vi "ReadSimbolValue.vi"(8 "error in (no error)":errorcluster, 10 "name":string, 11 "TCatAdsNet in":refnum<class "AdsNET.lvclass">) -> (0 "error out":errorcluster, 1 "Datatype":i32, 2 "Value":string, 3 "TCatAdsNet out":refnum<class "AdsNET.lvclass">, 4 "Elapsed Time (ms)":u32)   [LabVIEW 2016, in "TCatAdsNet.lvlib" / "AdsNET.lvclass"]
uses:
  AdsNET.lvclass
  AdsNET.lvclass/AdsNET.ctl
  C:/Users/Maurizio/Projects/twincat-lv-ads-library/TCatAdsNet Library/TwinCAT.Ads.dll
  TwinCAT.Ads.dll
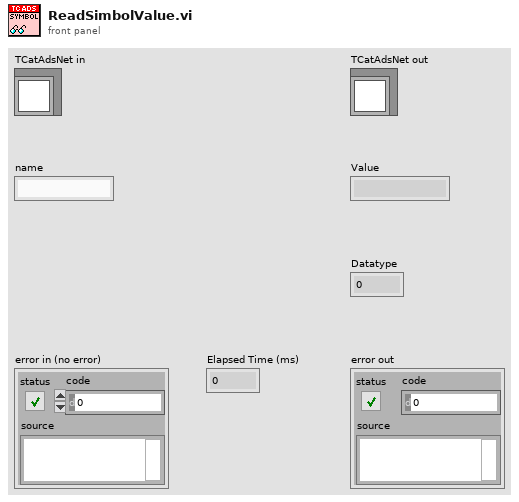
[diagram p1: front panel]
types:
  T1 = cluster{"Name":string, "IndexGroup":i64, "IndexOffset":i64, "Size":i32, "Type":string, "Datatype":i32, "Comment":string}
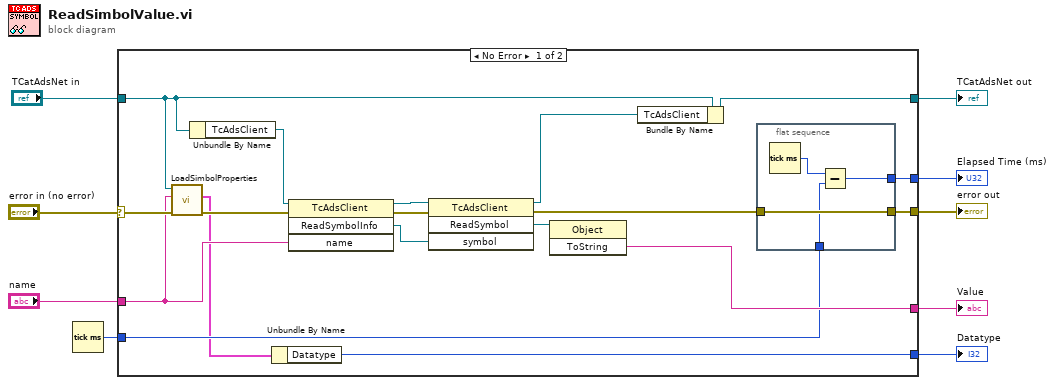
[diagram p0: block diagram]
diagram:
  n1 = Tick Count (ms)() -> (millisecond timer value=w3:u32)
  n2 = case shown="No Error" "error in (no error)" {
    selector: "error in (no error)" -> [w15 w32]
    tunnel: [w18 w32] -> w9
    tunnel: "TCatAdsNet in" -> [w12 w33]
    tunnel: "name" -> [w13 _]
    tunnel: [w22 _] -> w6
    tunnel: [w21 w33] -> w5
    tunnel: w3 -> [w17 _]
    tunnel: [w16 _] -> w2
    tunnel: [w10 _] -> w1
    frame No Error {
      n3 = call "LoadSimbolProperties.vi"("error in (no error)"=w15, "name"=w13, "TCatAdsNet in"=w12) -> ("error out"=w14:errorcluster, "SymbolProperties"=w11:T1)  [unwired: 5 in, 2 out]
      n4 = Unbundle By Name(w12) -> ("TcAdsClient"=w23:refnum<k24>)
      n5 = Unbundle By Name(w11) -> ("Datatype"=w10:i32)
      n6 = invoke class="TcAdsClient" method="ReadSymbolInfo"(reference=w23, error in=w14, "name"=w13) -> (reference out=w26:refnum<k24>, error out=w25:errorcluster, "ReadSymbolInfo"=w24:refnum<k24>)  [unwired: 1 in, 1 out]
      n7 = invoke class="TcAdsClient" method="ReadSymbol"(reference=w26, error in=w25, "symbol"=w24) -> (reference out=w20:refnum<k24>, error out=w19:errorcluster, "ReadSymbol"=w27:refnum<k24>)  [unwired: 1 in, 1 out]
      n8 = invoke class="Object" method="ToString"(reference=w27) -> ("ToString"=w22:string)  [unwired: 2 in, 2 out]
      n9 = Bundle By Name(cluster=w12, "TcAdsClient"=w20) -> (w21:refnum<class "AdsNET.lvclass">)
      n10 = flat-sequence {
        tunnel: w19 -> [w31]
        tunnel: [w31] -> w18
        tunnel: w17 -> [w29]
        tunnel: [w28] -> w16
        frame #0 {
          n11 = Tick Count (ms)() -> (millisecond timer value=w30:u32)
          n12 = Subtract(x=w30, y=w29) -> (x-y=w28:u32)
        }
      }
    }
    frame Error {
    }
  }
  "TCatAdsNet out" <- w5
  "error out" <- w9
  "Value" <- w6
  "Elapsed Time (ms)" <- w2
  "Datatype" <- w1
